vi "error handler.vi"(8 "error in (no error)":errorcluster, 11 "Next State in":T1) -> (0 "error out":errorcluster, 3 "Next State out":T1)   [LabVIEW 2013]
uses:
  Controls/StateMachineStates 1.ctl
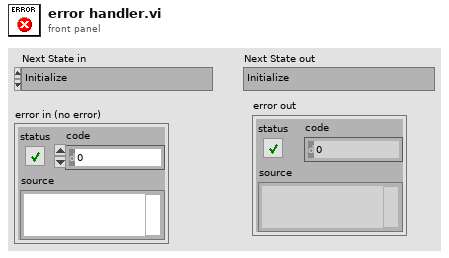
[diagram p1: front panel]
types:
  T1 = typedef "StateMachineStates 1.ctl" = enum16{"Initialize", "Idle", "determine next test case", "Set Dimmer", "Stabilize and Measure", "notify operator", "Stop"}
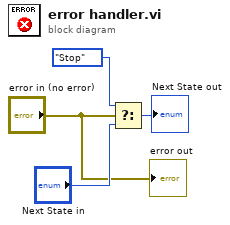
[diagram p0: block diagram]
diagram:
  n1 = Select(t=StateMachineStates_1."Stop", s="error in (no error)", f="Next State in") -> (s? t:f=→"Next State out":T1)
  "error out" <- "error in (no error)"
